vi "Initialize New Target.vi"(6 "instVIref":T1, 8 "tsRef":refnum<vi>) -> (3 "target out":refnum<class "Base Target.lvclass">)   [LabVIEW 2020, in "NI_TargetHelper.lvlib"]
uses:
  <vilib>/TargetSupport/NI_TargetHelper/NI_TargetHelper.lvlib
  <vilib>/TargetSupport/NI_TargetHelper/Base Target/Base Target.lvclass
  <vilib>/TargetSupport/NI_TargetHelper/Instance VIref.ctl
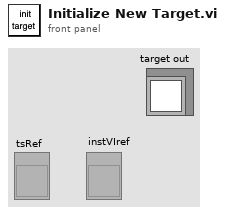
[diagram p1: front panel]
types:
  T1 = typedef "NI_TargetHelper.lvlib/Instance VIref.ctl" = refnum<vi>
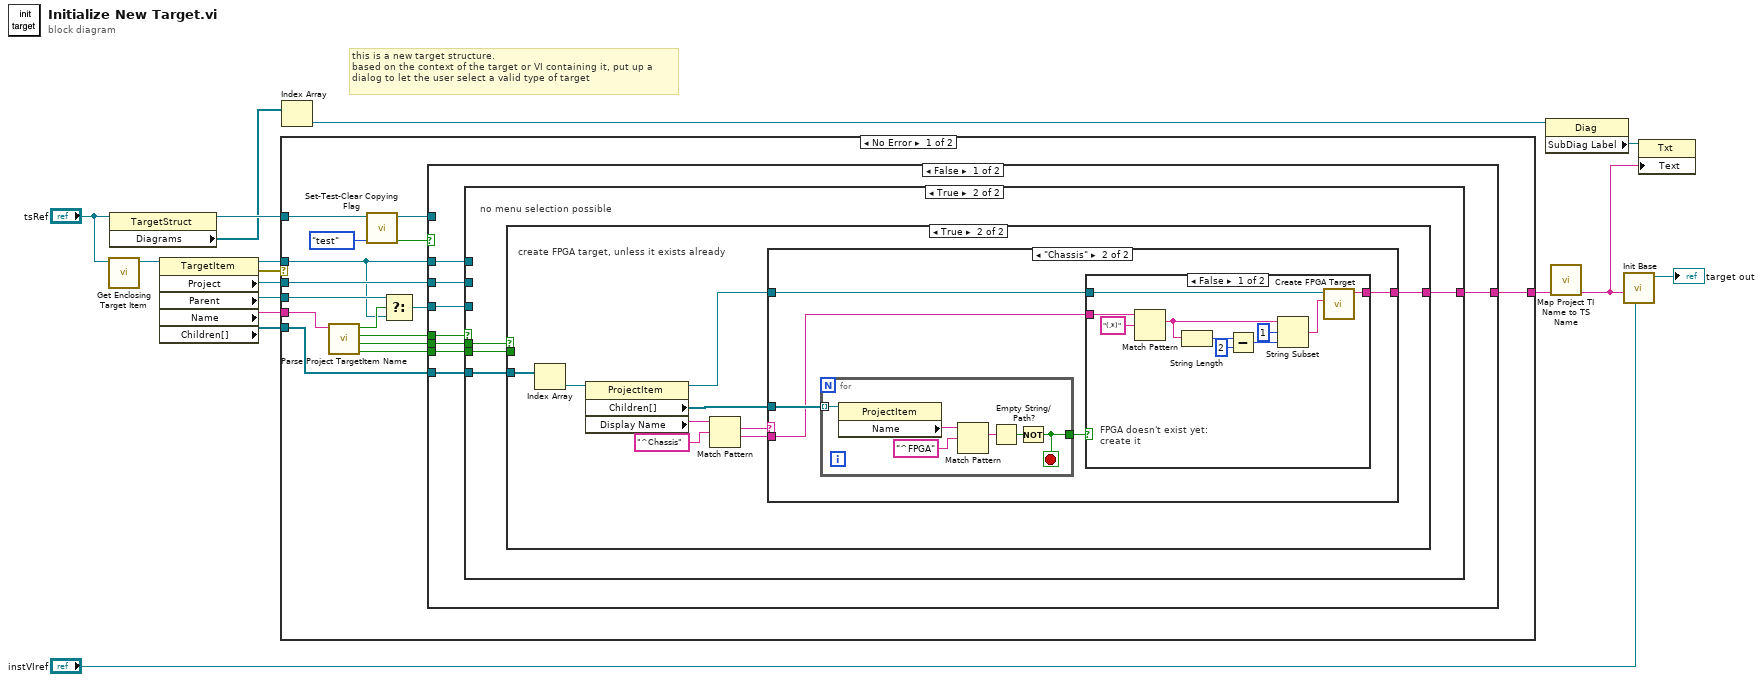
[diagram p0: block diagram]
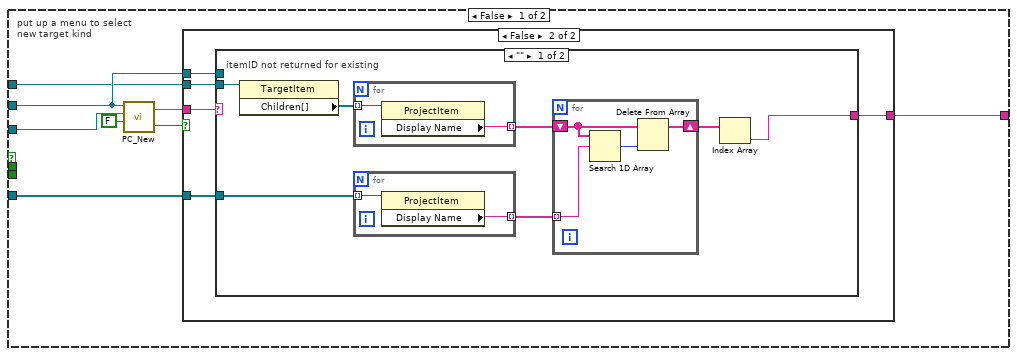
[diagram p2: hidden frame]
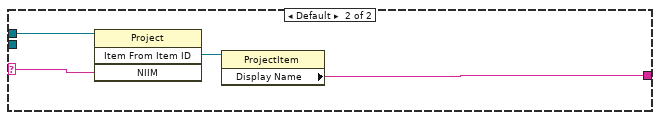
[diagram p4: hidden frame]
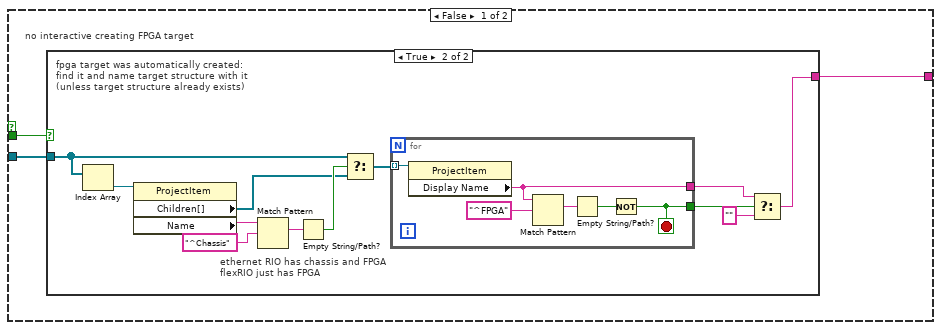
[diagram p5: hidden frame]
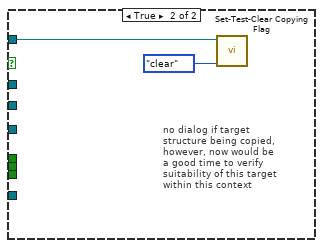
[diagram p9: hidden frame]
diagram:
  # "this is a new target structure.\nbased on the context of the target or VI containing it, put up a\ndialog to let the user select a valid type of target"
  n1 = call <vilib>:"Get Enclosing Target Item.vi"("tsRef"="tsRef") -> ("targetItem"=w4:refnum<vi>)  [unwired: 10 in]
  n2 = property class="TargetStruct"(reference="tsRef") -> (reference out=w3:refnum<vi>, "Diagrams"=w2:refnum<vi>[])  [unwired: 1 in, 1 out]
  n3 = property class="TargetItem"(reference=w4) -> (reference out=w12:refnum<vi>, error out=w13:errorcluster, "Project"=w14:refnum<vi>, "Parent"=w11:refnum<vi>, "Name"=w10:string, "Children[]"=w5:refnum<vi>[])  [unwired: 1 in]
  n4 = case shown="No Error" w13 {
    tunnel: w14 -> [w31 _]
    tunnel: [w30 _] -> w9
    tunnel: w3 -> [w29 _]
    tunnel: w12 -> [w17 _]
    tunnel: w5 -> [w18 _]
    tunnel: w11 -> [w25 _]
    tunnel: w10 -> [w23 _]
    frame No Error {
      n5 = call <vilib>:"Parse Project TargetItem Name.vi"("project targetitem name"=w23) -> ("find fpga & create target struct, unless exists already"=w19:bool, "create fpga, unless exists already"=w20:bool, "no menu"=w21:bool, "use owner menu"=w22:bool)  [unwired: 7 in]
      n6 = call <vilib>:"Set-Test-Clear Copying Flag.vi"("op"=enum16{"test", "clear", "set"}."test", "tsRef"=w29) -> ("copying"=w28:bool, "tsRef out"=w26:refnum<vi>)  [unwired: 8 in]
      n7 = Select(t=w25, s=w22, f=w17) -> (s? t:f=w24:refnum<vi>)
      n8 = case shown="False" w28 {
        tunnel: w31 -> [w37 _]
        tunnel: w24 -> [w39 _]
        tunnel: [w38 _] -> w30
        tunnel: w26 -> [_ w127]
        tunnel: w21 -> [w36 _]
        tunnel: w20 -> [w35 _]
        tunnel: w19 -> [w34 _]
        tunnel: w18 -> [w33 _]
        tunnel: w17 -> [w32 _]
        frame False {
          n9 = case shown="True" w36 {
            tunnel: w39 -> [w46 _]
            tunnel: [w45 w72] -> w38
            tunnel: w37 -> [w44 _]
            tunnel: w35 -> [_ w75]
            tunnel: w34 -> [_ w74]
            tunnel: w33 -> [w40 w73]
            tunnel: w32 -> [w41 _]
            frame False {
              # "put up a menu to select \nnew target kind"
              n10 = call <resource>:"PC_New.vi"("EnableMultiselect"=FALSE, "Item"=w46, "Project"=w44) -> ("Canceled?"=w42:bool, "Item ID"=w43:string)  [unwired: 1 in]
              n11 = case shown="False" w42 {
                tunnel: [_ w50] -> w45
                tunnel: w44 -> [_ w52]
                tunnel: w43 -> [_ w51]
                tunnel: w41 -> [_ w49]
                tunnel: w40 -> [_ w48]
                frame True {
                  # "cancellation makes generic target"
                }
                frame False {
                  n12 = case shown="\"\"" w51 {
                    selector: w51 -> [_ w70]
                    tunnel: w52 -> [_ w71]
                    tunnel: [w53 w68] -> w50
                    tunnel: w49 -> [w59 _]
                    tunnel: w48 -> [w57 _]
                    frame "" {
                      # "itemID not returned for existing"
                      n13 = property class="TargetItem"(reference=w59) -> ("Children[]"=w58:refnum<vi>[])  [unwired: 1 in, 2 out]
                      n14 = for {
                        tunnel: w58 -> [w63] mode=indexing
                        tunnel: [w62] -> w56 mode=indexing
                        n15 = property class="ProjectItem"(reference=w63) -> ("Display Name"=w62:string)  [unwired: 1 in, 2 out]
                      }
                      n16 = for {
                        tunnel: w57 -> [w61] mode=indexing
                        tunnel: [w60] -> w55 mode=indexing
                        n17 = property class="ProjectItem"(reference=w61) -> ("Display Name"=w60:string)  [unwired: 1 in, 2 out]
                      }
                      n18 = for {
                        tunnel: w55 -> [w64] mode=indexing
                        shift-right: [w65] -> w54
                        shift-left: w56 -> [w66]
                        n19 = Search 1D Array(1D array=w66, element=w64) -> (index of element=w67:i32)  [unwired: 1 in]
                        n20 = Delete From Array(array=w66, index=w67) -> (array with subset deleted=w65:string[])  [unwired: 1 in, 1 out]
                      }
                      n21 = Index Array(array=w54) -> (element=w53:string)  [unwired: 1 in]
                    }
                    frame Default {
                      n22 = invoke class="Project" method="Item From Item ID"(reference=w71, "NIIM"=w70) -> ("GetItemFromNIIM"=w69:refnum<vi>)  [unwired: 2 in, 3 out]
                      n23 = property class="ProjectItem"(reference=w69) -> ("Display Name"=w68:string)  [unwired: 1 in, 2 out]
                    }
                  }
                }
              }
            }
            frame True {
              # "no menu selection possible"
              n24 = case shown="True" w75 {
                tunnel: w74 -> [w78 _]
                tunnel: w73 -> [w76 w105]
                tunnel: [w77 w99] -> w72
                frame False {
                  # "no interactive creating FPGA target"
                  n25 = case shown="True" w78 {
                    tunnel: [_ w79] -> w77
                    tunnel: w76 -> [_ w85]
                    frame False {
                      # "what's going on?"
                    }
                    frame True {
                      # "ethernet RIO has chassis and FPGA\nflexRIO just has FPGA"
                      # "fpga target was automatically created:\nfind it and name target structure with it\n(unless target structure already exists)"
                      n26 = Index Array(array=w85) -> (element=w90:refnum<vi>)  [unwired: 1 in]
                      n27 = property class="ProjectItem"(reference=w90) -> ("Children[]"=w84:refnum<vi>[], "Name"=w89:string)  [unwired: 1 in, 2 out]
                      n28 = Match Pattern(string=w89, regular expression="^Chassis") -> (match substring=w87:string)  [unwired: 1 in, 3 out]
                      n29 = Empty String/Path?(string/path=w87) -> (empty?=w86:bool)
                      n30 = Select(t=w85, s=w86, f=w84) -> (s? t:f=w83:refnum<vi>[])
                      n31 = for {
                        tunnel: w83 -> [w96] mode=indexing
                        tunnel: [w91] -> w82
                        tunnel: [w94] -> w81
                        stop <- w91 stop-if-true
                        n32 = property class="ProjectItem"(reference=w96) -> ("Display Name"=w94:string)  [unwired: 1 in, 2 out]
                        n33 = Match Pattern(string=w94, regular expression="^FPGA") -> (match substring=w93:string)  [unwired: 1 in, 3 out]
                        n34 = Empty String/Path?(string/path=w93) -> (empty?=w92:bool)
                        n35 = Not(x=w92) -> (.not. x?=w91:bool)
                      }
                      n36 = Select(t=w81, s=w82, f="") -> (s? t:f=w79:string)
                    }
                  }
                }
                frame True {
                  # "create FPGA target, unless it exists already"
                  n37 = Index Array(array=w105) -> (element=w104:refnum<vi>)  [unwired: 1 in]
                  n38 = property class="ProjectItem"(reference=w104) -> (reference out=w97:refnum<vi>, "Children[]"=w100:refnum<vi>[], "Display Name"=w101:string)  [unwired: 1 in, 1 out]
                  n39 = Match Pattern(string=w101, regular expression="^Chassis") -> (match substring=w102:string, after substring=w98:string)  [unwired: 1 in, 2 out]
                  n40 = case shown="\"Chassis\"" w102 {
                    tunnel: w100 -> [_ w110]
                    tunnel: [_ w108] -> w99
                    tunnel: w98 -> [_ w107]
                    tunnel: w97 -> [_ w106]
                    frame Default {
                      # "what's going on?"
                    }
                    frame "Chassis" {
                      n41 = for {
                        tunnel: w110 -> [w126] mode=indexing
                        tunnel: [w121] -> w109
                        stop <- w121 stop-if-true
                        n42 = property class="ProjectItem"(reference=w126) -> ("Name"=w125:string)  [unwired: 1 in, 2 out]
                        n43 = Match Pattern(string=w125, regular expression="^FPGA") -> (match substring=w122:string)  [unwired: 1 in, 3 out]
                        n44 = Empty String/Path?(string/path=w122) -> (empty?=w123:bool)
                        n45 = Not(x=w123) -> (.not. x?=w121:bool)
                      }
                      n46 = case shown="False" w109 {
                        tunnel: [w120 _] -> w108
                        tunnel: w107 -> [w119 _]
                        tunnel: w106 -> [w111 _]
                        frame False {
                          # "FPGA doesn't exist yet:\ncreate it"
                          n47 = Match Pattern(string=w119, regular expression="(.*)") -> (match substring=w116:string)  [unwired: 1 in, 3 out]
                          n48 = String Length(string=w116) -> (length=w115:i32)
                          n49 = Subtract(x=w115, y=2) -> (x-y=w113:i32)
                          n50 = String Subset(string=w116, offset (0)=1, length (rest)=w113) -> (substring=w112:string)
                          n51 = call <vilib>:"Create FPGA Target.vi"("target class"=w112, "Parent Item In"=w111) -> ("target structure name"=w120:string)  [unwired: 9 in]
                        }
                        frame True {
                          # "FPGA already exists:\njust create a new generic target"
                        }
                      }
                    }
                  }
                }
              }
            }
          }
        }
        frame True {
          # "no dialog if target \nstructure being copied,\nhowever, now would be\na good time to verify\nsuitability of this target\nwithin this context"
          n52 = call <vilib>:"Set-Test-Clear Copying Flag.vi"("op"=enum16{"test", "clear", "set"}."clear", "tsRef"=w127) -> ()  [unwired: 8 in, 2 out]
        }
      }
    }
    frame Error {
    }
  }
  n53 = Index Array(array=w2) -> (element=w16:refnum<vi>)  [unwired: 1 in]
  n54 = property class="Diag"(reference=w16) -> ("SubDiag Label"=w15:refnum<vi>)  [unwired: 1 in, 2 out]
  n55 = call <vilib>:"Map Project TI Name to TS Name.vi"("project targetitem name"=w9) -> ("target structure name"=w8:string)  [unwired: 10 in]
  n56 = call <vilib>:"Init Base.vi"("instVIref"="instVIref", "target structure name"=w8) -> ("target out"=→"target out":refnum<class "Base Target.lvclass">)  [unwired: 9 in]
  n57 = property class="Txt"(reference=w15, "Text"=w8) -> ()  [unwired: 1 in, 2 out]
